vi "Dispose.vi"(8 "error in (no error)":errorcluster, 11 "Pub Sub Message Channel in":refnum<class "Pub Sub Message Channel.lvclass">) -> (0 "error out":errorcluster, 3 "Pub Sub Message Channel in 2":refnum<class "Pub Sub Message Channel.lvclass">)   [LabVIEW 2020, in "Actor Pub Sub Channels.lvlib" / "Pub Sub Message Channel.lvclass"]
uses:
  Pub Sub Message Channel.lvclass
  Pub Sub Message Channel.lvclass/Pub Sub Message Channel.ctl
  <vilib>/ActorFramework/Message Queue/Message Queue.lvclass
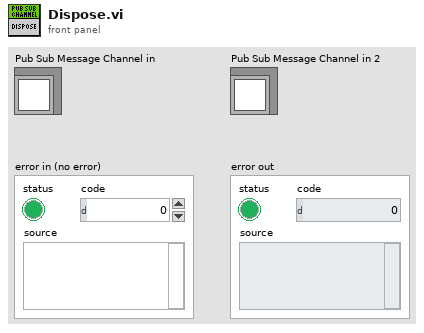
[diagram p1: front panel]
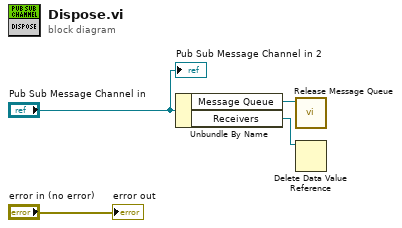
[diagram p0: block diagram]
diagram:
  n1 = Unbundle By Name("Pub Sub Message Channel in") -> ("Message Queue"=w2:refnum<class "Message Queue.lvclass">, "Receivers"=w1:refnum<data-value>)
  n2 = call <vilib>:"Release Message Queue.vi"("Message Queue"=w2) -> ()  [unwired: 9 in, 2 out]
  n3 = Delete Data Value Reference(data value reference=w1) -> ()  [unwired: 1 in, 2 out]
  "Pub Sub Message Channel in 2" <- "Pub Sub Message Channel in"
  "error out" <- "error in (no error)"
